vi "setIndex.vi"(8 "error in (no error)":errorcluster, 10 "index":cluster{"row":i32, "column":i32}, 11 "SudukuState in":refnum<class "SudukuState.lvclass">) -> (0 "error out":errorcluster, 3 "SudukuState out":refnum<class "SudukuState.lvclass">)   [LabVIEW 2009]
uses:
  SudukuState.lvclass
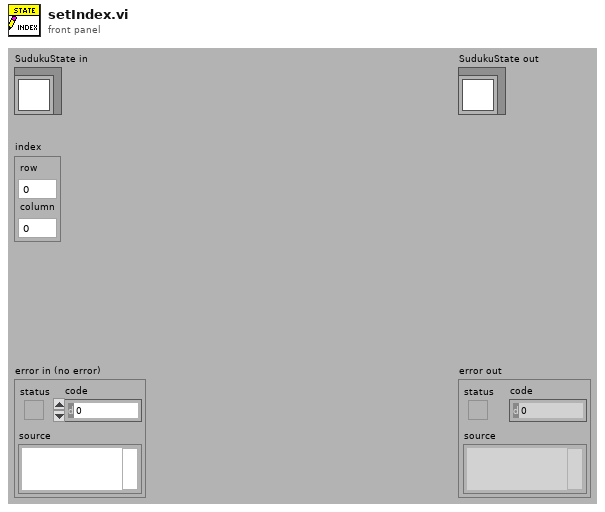
[diagram p1: front panel]
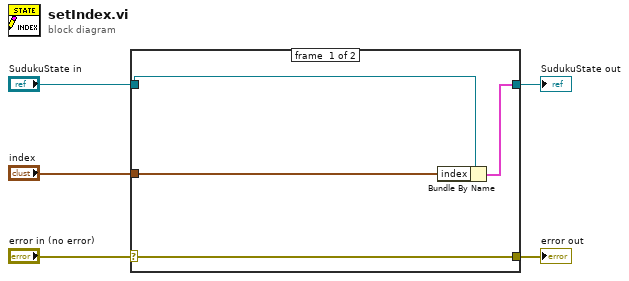
[diagram p0: block diagram]
diagram:
  n1 = case shown="No Error" "error in (no error)" {
    selector: "error in (no error)" -> [w9 w10]
    tunnel: [w9 w10] -> w4
    tunnel: [w7 w11] -> w2
    tunnel: "SudukuState in" -> [w8 w11]
    tunnel: "index" -> [w6 _]
    frame #0 {
      n2 = Bundle By Name(cluster=w8, "index"=w6) -> (w7:cluster{})
    }
    frame #1 {
    }
  }
  "error out" <- w4
  "SudukuState out" <- w2
